vi "USB6343_Control_v1.4.vi"   [LabVIEW 2013]
uses:
  <vilib>/DAQmx/read.llb/DAQmx Read (Digital 1D Bool NChan 1Samp 1Line).vi
  <vilib>/DAQmx/read.llb/DAQmx Read (Analog 1D DBL NChan 1Samp).vi
  <vilib>/DAQmx/miscellaneous.llb/DAQmx Fill In Error Info.vi
  <vilib>/DAQmx/configure/timing.llb/DAQmx Timing (Implicit).vi
  offsets.vi
  <vilib>/DAQmx/write.llb/DAQmx Write (Digital 1D Bool NChan 1Samp 1Line).vi
  <vilib>/DAQmx/write.llb/DAQmx Write (Analog 1D DBL NChan 1Samp).vi
types:
  T1 = cluster{"source":string, "channel":i32, "old value":dbl, "new value":dbl, "on/off":bool}
  T2 = cluster{"cmd":string, "channel":i32, "value":dbl, "on/off":bool, "return value":refnum<vi>}
  T3 = cluster{"AI Task":refnum<k21>, "AO Task":refnum<k21>, "DO Task":refnum<k21>, "DI Task":refnum<k21>, "PWM x":refnum<k21>, "PWM y":refnum<k21>, "counter x":refnum<k21>, "counter y":refnum<k21>}
  T4 = cluster{"data":dbl, "data":dbl, "data":dbl, "data":dbl}
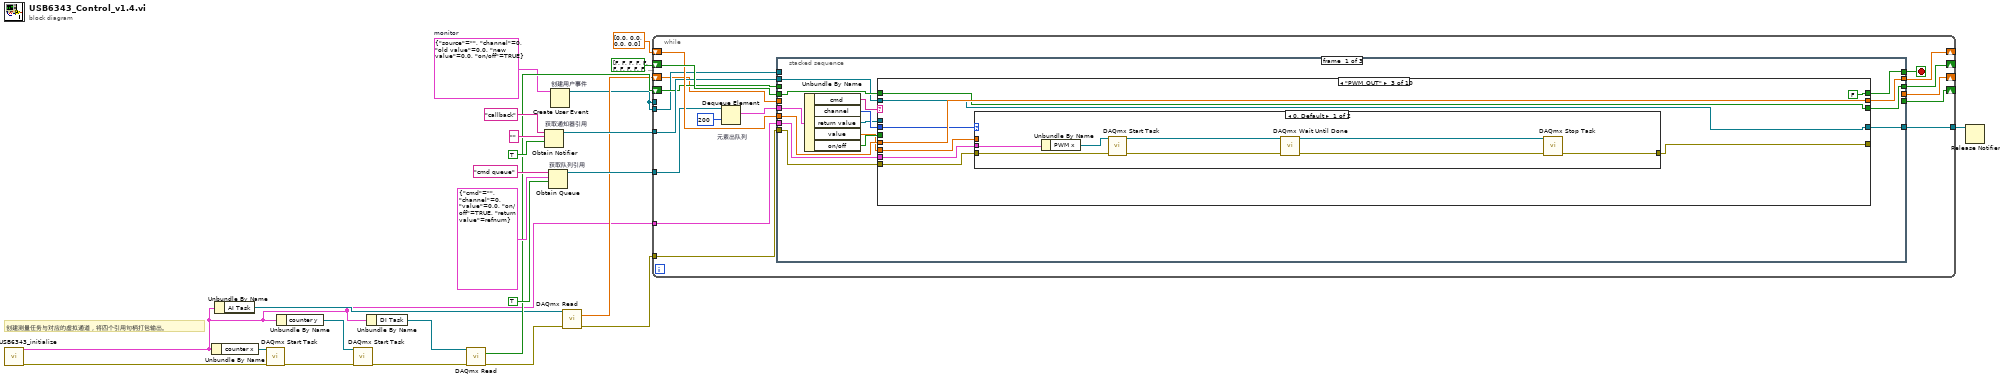
[diagram p0: block diagram]
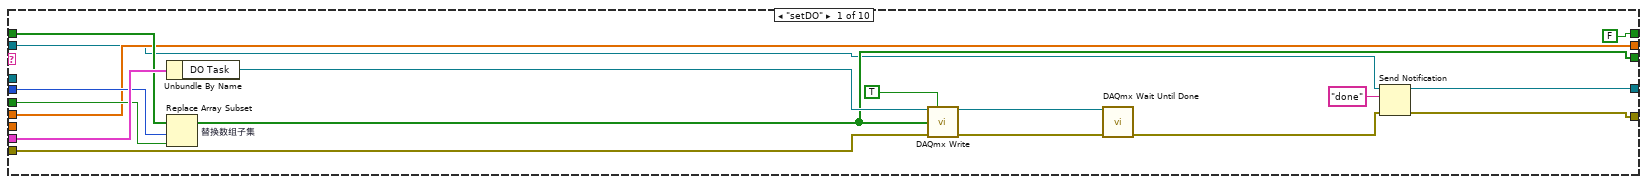
[diagram p2: hidden frame]
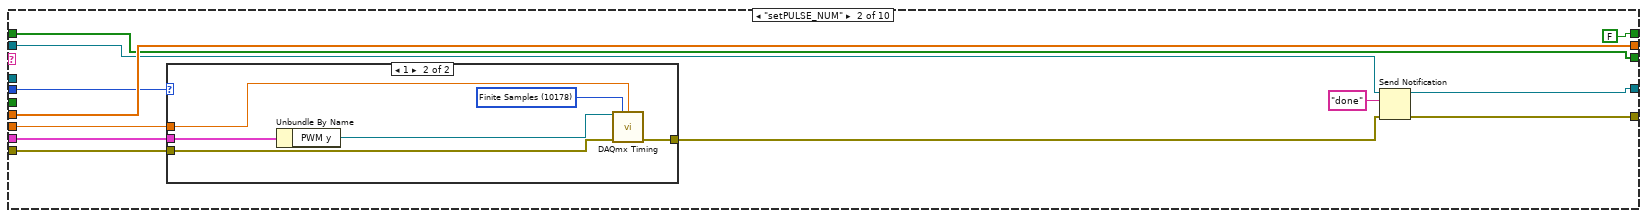
[diagram p3: hidden frame]
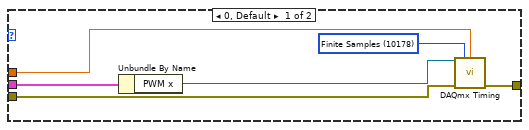
[diagram p4: hidden frame]
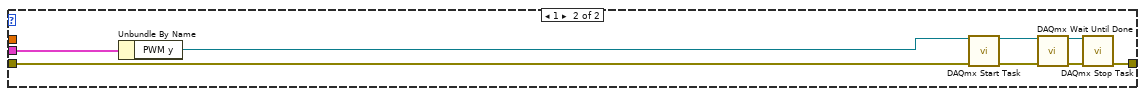
[diagram p5: hidden frame]
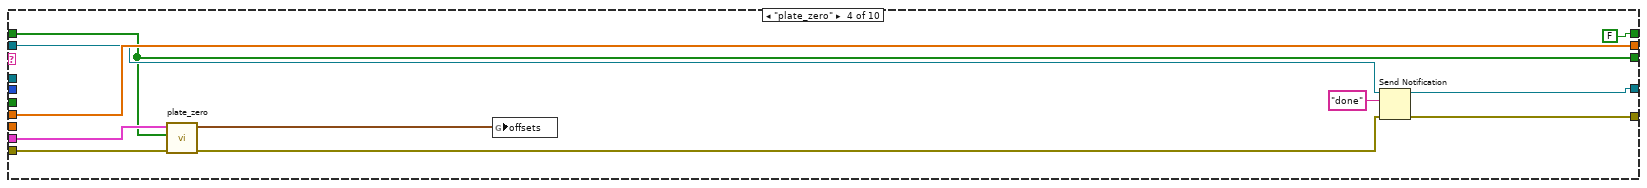
[diagram p6: hidden frame]
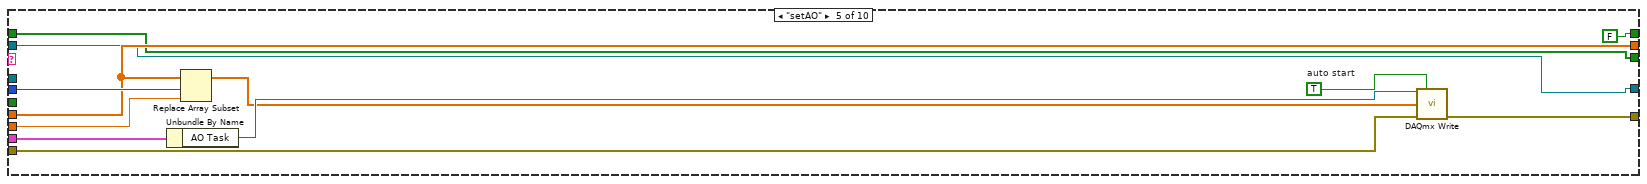
[diagram p7: hidden frame]
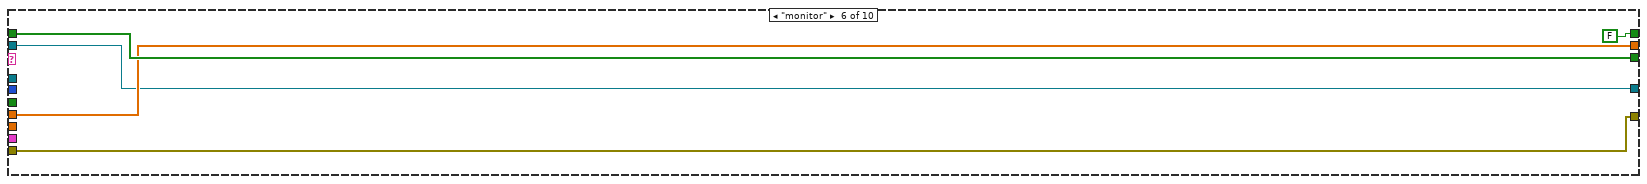
[diagram p8: hidden frame]
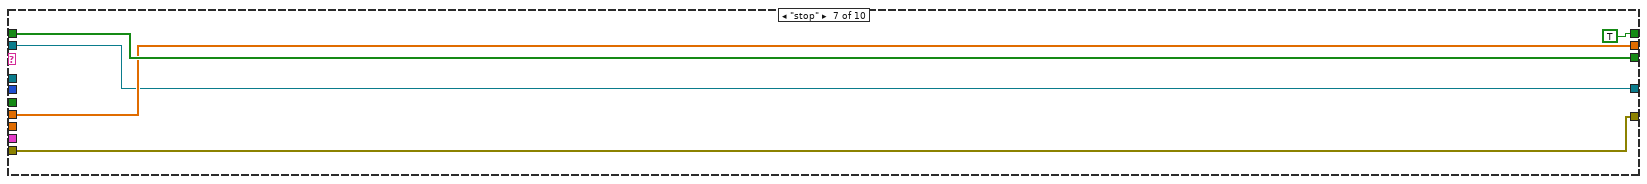
[diagram p9: hidden frame]
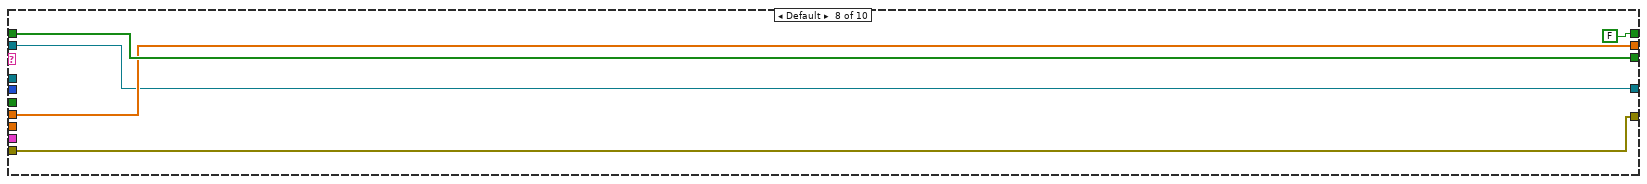
[diagram p10: hidden frame]
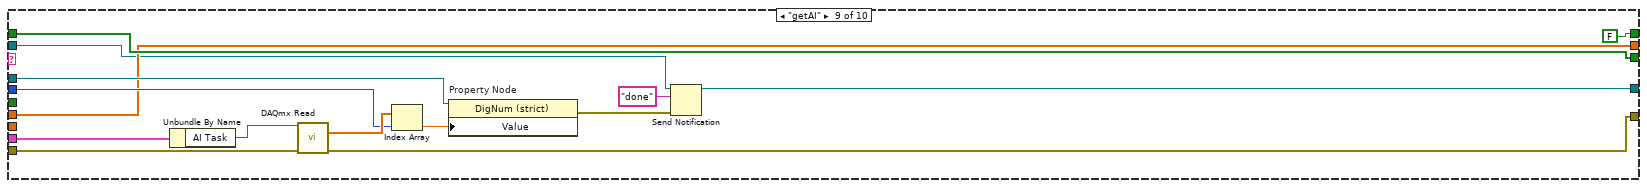
[diagram p11: hidden frame]
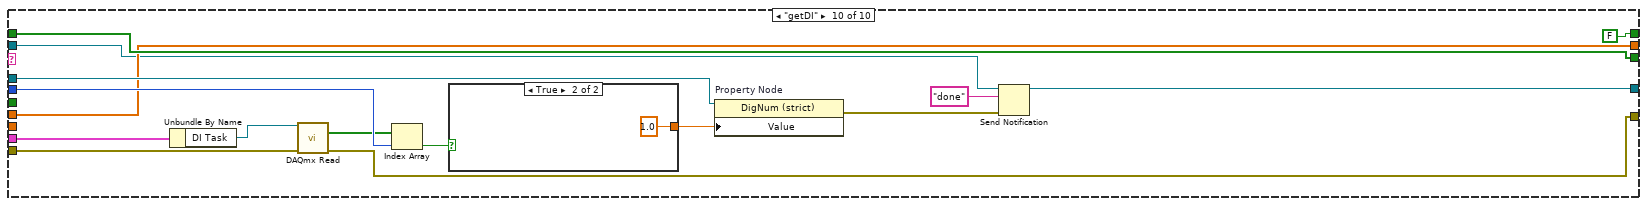
[diagram p12: hidden frame]
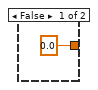
[diagram p13: hidden frame]
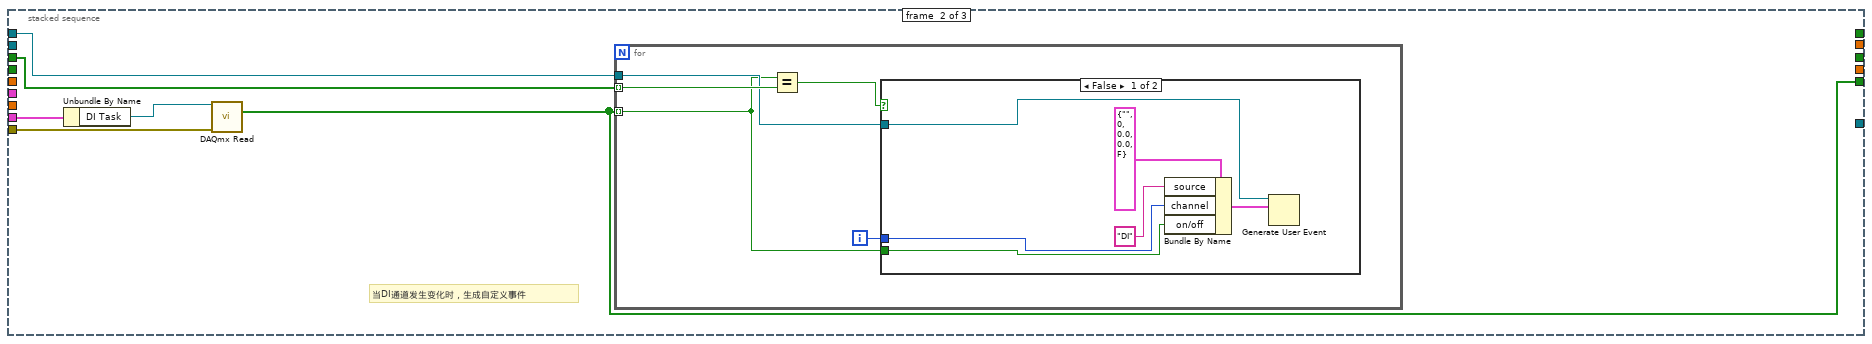
[diagram p14: hidden frame]
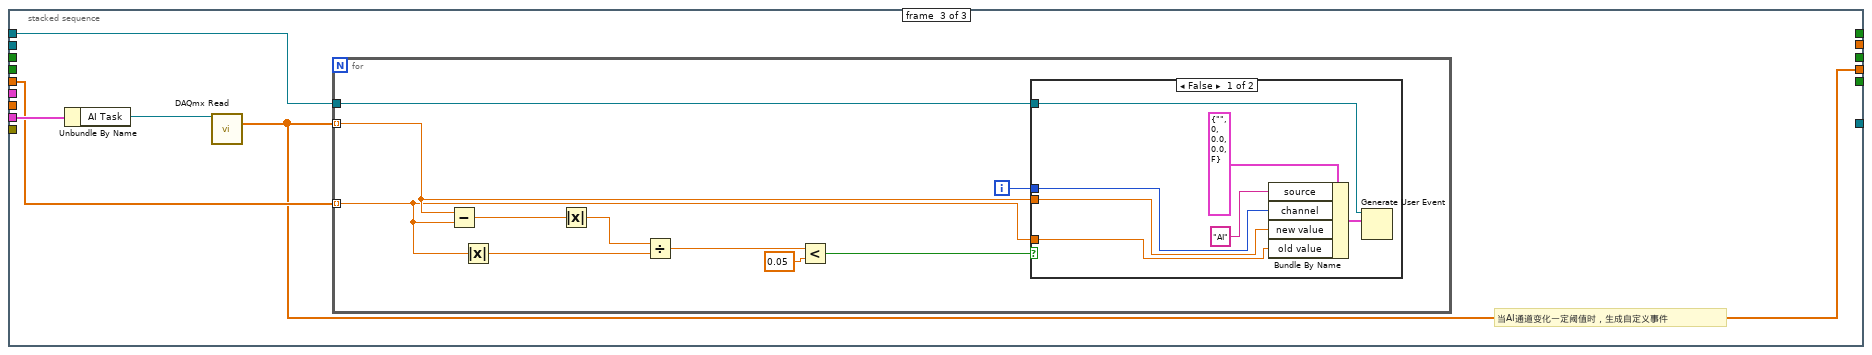
[diagram p16: hidden frame]
diagram:
  w8 = T1 {"source"="", "channel"=0, "old value"=0.0, "new value"=0.0, "on/off"=TRUE}  # monitor
  # "创建测量任务与对应的虚拟通道，将四个引用句柄打包输出。"
  n1 = call "USB6343_initialize.vi"() -> ("error out"=w5:errorcluster, "tasks"=w2:T3)  [unwired: 10 in]
  n2 = Unbundle By Name(w2) -> ("counter x"=w3:refnum<k21>)
  n3 = Unbundle By Name(w2) -> ("AI Task"=w10:refnum<k21>)
  n4 = call <vilib>:"DAQmx Start Task.vi"("task/channels in"=w3, "error in"=w5) -> ("error out"=w6:errorcluster)  [unwired: 12 in, 1 out]
  n5 = Unbundle By Name(w2) -> ("counter y"=w1:refnum<k21>)
  n6 = call <vilib>:"DAQmx Start Task.vi"("task/channels in"=w1, "error in"=w6) -> ("error out"=w4:errorcluster)  [unwired: 12 in, 1 out]
  n7 = Unbundle By Name(w2) -> ("DI Task"=w14:refnum<k21>)
  n8 = call-poly <vilib>:"DAQmx Read.vi"("task/channels in"=w14, "error in"=w4) -> ("data"=w13:bool[], "error out"=w12:errorcluster)  [unwired: 11 in, 1 out]
  n9 = Obtain Notifier "获取通知器引用"(name (unnamed)="callback" ("名称（未命名）"), notification data type="", create if not found? (T)=TRUE ("如未找到是否创建？(T)")) -> (notifier out=w17:refnum<notifier>)  [unwired: 1 in, 2 out]
  n10 = Obtain Queue "获取队列引用"(name (unnamed)="cmd queue" ("名称（未命名）"), element data type=T2 {"cmd"="", "channel"=0, "value"=0.0, "on/off"=TRUE, "return value"=refnum}, create if not found? (T)=TRUE ("如未找到是否创建？(T)")) -> (queue out=w21:refnum<queue>)  [unwired: 2 in, 2 out]
  n11 = Create User Event "创建用户事件"(user event datatype=w8) -> (user event=w7:refnum<user-event>)  [unwired: 1 in, 1 out]
  n12 = call-poly <vilib>:"DAQmx Read.vi"("task/channels in"=w10, "error in"=w12) -> ("data"=w9:dbl[], "error out"=w11:errorcluster)  [unwired: 11 in, 1 out]
  n13 = while {
    tunnel: w2 -> [w36]
    tunnel: w11 -> [w42]
    shift-right: [w40] -> _
    shift-left: bool[] [FALSE, FALSE, FALSE, FALSE, FALSE, FALSE, FALSE, FALSE, FALSE, FALSE, FALSE, FALSE, FALSE, FALSE, FALSE, FALSE] -> [w41]
    shift-right: [w37] -> _
    shift-left: dbl[] [0.0, 0.0, 0.0, 0.0] ("data") -> [w38]
    tunnel: w21 -> [w35]
    tunnel: w17 -> [w32]
    tunnel: [w31] -> w16
    shift-right: [w29] -> _
    shift-left: w13 -> [w30]
    shift-right: [w26] -> _
    shift-left: w9 -> [w27]
    tunnel: w7 -> [w28]
    tunnel: w7 -> [_]
    stop <- w39 stop-if-true
    n14 = Dequeue Element "元素出队列"(queue=w35, timeout in ms (-1)=200 ("超时毫秒(-1)")) -> (element=w34:T2)  [unwired: 1 in, 3 out]
    n15 = stacked-sequence {
      tunnel: w42 -> [w57 w198 _]
      tunnel: w41 -> [w56 _ _]
      tunnel: [w55 _ _] -> w40
      tunnel: [w54 _ _] -> w39
      tunnel: w38 -> [w53 _ _]
      tunnel: [w52 _ _] -> w37
      tunnel: w36 -> [w43 w200 w216]
      tunnel: w34 -> [w51 _ _]
      tunnel: w32 -> [w45 _ _]
      tunnel: [w44 _ _] -> w31
      tunnel: w30 -> [_ w197 _]
      tunnel: [_ w196 _] -> w29
      tunnel: w28 -> [_ w195 w212]
      tunnel: w27 -> [_ _ w214]
      tunnel: [_ _ w213] -> w26
      frame #0 {
        n16 = Unbundle By Name(w51) -> ("cmd"=w50:string, "channel"=w49:i32, "return value"=w48:refnum<vi>, "value"=w46:dbl, "on/off"=w47:bool)
        n17 = case shown="\"PWM_OUT\"" w50 {
          tunnel: w49 -> [w72 w75 w101 _ w144 _ _ _ w171 w190]
          tunnel: w43 -> [w74 w79 w104 w128 w146 _ _ _ w176 w192]
          tunnel: w57 -> [w66 w77 w102 w126 w138 w148 w153 w158 w173 w182]
          tunnel: w56 -> [w73 w80 w105 w127 w142 w151 w156 w161 w169 w189]
          tunnel: w47 -> [w71 _ _ _ _ _ _ _ _ _]
          tunnel: [w64 w80 w105 w127 w142 w151 w156 w161 w169 w189] -> w55
          tunnel: [FALSE FALSE FALSE FALSE FALSE FALSE TRUE FALSE FALSE FALSE] -> w54
          tunnel: w53 -> [w69 w85 w106 w133 w143 w150 w154 w159 w168 w188]
          tunnel: [w69 w85 w106 w133 w143 w150 w154 w159 w168 w188] -> w52
          tunnel: w48 -> [_ _ _ _ _ _ _ _ w174 w191]
          tunnel: [w68 w84 w100 w132 w135 w148 w153 w158 w166 w181] -> _
          tunnel: w46 -> [_ w78 w103 _ w137 _ _ _ _ _]
          tunnel: w45 -> [w59 w82 w99 w131 w136 w147 w152 w157 w163 w184]
          tunnel: [w58 w81 w99 w130 w136 w147 w152 w157 w162 w183] -> w44
          frame "setDO" {
            n18 = Unbundle By Name(w74) -> ("DO Task"=w65:refnum<k21>)
            n19 = Replace Array Subset "替换数组子集"(array=w73, new element=w71, index=w72) -> (w64:bool[])
            n20 = call-poly <vilib>:"DAQmx Write.vi"("task/channels in"=w65, "auto start"=TRUE, "data"=w64, "error in"=w66) -> ("task out"=w60:refnum<k21>, "error out"=w62:errorcluster)  [unwired: 9 in, 1 out]
            n21 = call <vilib>:"DAQmx Wait Until Done.vi"("task/channels in"=w60, "error in"=w62) -> ("error out"=w61:errorcluster)  [unwired: 12 in, 1 out]
            n22 = Send Notification(notification="done" ("通知"), notifier=w59, error in (no error)=w61) -> (notifier out=w58:refnum<notifier>, error out=w68:errorcluster)
          }
          frame "setPULSE_NUM" {
            n23 = case shown="1" w75 {
              tunnel: w79 -> [w92 w98]
              tunnel: w78 -> [w89 w95]
              tunnel: w77 -> [w88 w94]
              tunnel: [w87 w93] -> w76
              frame 0, Default {
                w90 = 10178 items=["Finite Samples"=10178, "Continuous Samples"=10123, "Hardware Timed Single Point"=12522] ("sample mode")
                n24 = Unbundle By Name(w92) -> ("PWM x"=w91:refnum<k21>)
                n25 = call-poly <vilib>:"DAQmx Timing.vi"("task/channels in"=w91, "sample mode"=w90, "samples per channel"=w89, "error in"=w88) -> ("error out"=w87:errorcluster)  [unwired: 10 in, 1 out]
              }
              frame 1 {
                w96 = 10178 items=["Finite Samples"=10178, "Continuous Samples"=10123, "Hardware Timed Single Point"=12522] ("sample mode")
                n26 = Unbundle By Name(w98) -> ("PWM y"=w97:refnum<k21>)
                n27 = call-poly <vilib>:"DAQmx Timing.vi"("task/channels in"=w97, "sample mode"=w96, "samples per channel"=w95, "error in"=w94) -> ("error out"=w93:errorcluster)  [unwired: 10 in, 1 out]
              }
            }
            n28 = Send Notification(notification="done" ("通知"), notifier=w82, error in (no error)=w76) -> (notifier out=w81:refnum<notifier>, error out=w84:errorcluster)
          }
          frame "PWM_OUT" {
            n29 = case shown="0, Default" w101 {
              tunnel: w104 -> [w115 w123]
              tunnel: w103 -> [_ _]
              tunnel: w102 -> [w113 w121]
              tunnel: [w108 w116] -> w100
              frame 0, Default {
                n30 = Unbundle By Name(w115) -> ("PWM x"=w114:refnum<k21>)
                n31 = call <vilib>:"DAQmx Start Task.vi"("task/channels in"=w114, "error in"=w113) -> ("task out"=w111:refnum<k21>, "error out"=w112:errorcluster)  [unwired: 12 in]
                n32 = call <vilib>:"DAQmx Wait Until Done.vi"("task/channels in"=w111, "error in"=w112) -> ("task out"=w109:refnum<k21>, "error out"=w110:errorcluster)  [unwired: 12 in]
                n33 = call <vilib>:"DAQmx Stop Task.vi"("task/channels in"=w109, "error in"=w110) -> ("error out"=w108:errorcluster)  [unwired: 12 in, 1 out]
              }
              frame 1 {
                n34 = Unbundle By Name(w123) -> ("PWM y"=w122:refnum<k21>)
                n35 = call <vilib>:"DAQmx Start Task.vi"("task/channels in"=w122, "error in"=w121) -> ("task out"=w119:refnum<k21>, "error out"=w120:errorcluster)  [unwired: 12 in]
                n36 = call <vilib>:"DAQmx Wait Until Done.vi"("task/channels in"=w119, "error in"=w120) -> ("task out"=w117:refnum<k21>, "error out"=w118:errorcluster)  [unwired: 12 in]
                n37 = call <vilib>:"DAQmx Stop Task.vi"("task/channels in"=w117, "error in"=w118) -> ("error out"=w116:errorcluster)  [unwired: 12 in, 1 out]
              }
            }
          }
          frame "plate_zero" {
            n38 = call "plate_zero.vi"("error in"=w126, "DO array"=w127, "tasks"=w128) -> ("error out"=w125:errorcluster, "offsets"=w124:T4)  [unwired: 7 in]
            n39 = global write "offsets.vi" "offsets"(w124) -> ()
            n40 = Send Notification(notification="done", notifier=w131, error in (no error)=w125) -> (notifier out=w130:refnum<notifier>, error out=w132:errorcluster)
          }
          frame "setAO" {
            w140 = TRUE  # auto start
            n41 = Unbundle By Name(w146) -> ("AO Task"=w145:refnum<k21>)
            n42 = Replace Array Subset(array=w143, new element=w137, index=w144) -> (w141:dbl[])
            n43 = call-poly <vilib>:"DAQmx Write.vi"("task/channels in"=w145, "auto start"=w140, "data"=w141, "error in"=w138) -> ("error out"=w135:errorcluster)  [unwired: 9 in, 2 out]
          }
          frame "monitor" {
          }
          frame "stop" {
          }
          frame Default {
          }
          frame "getAI" {
            n44 = Unbundle By Name(w176) -> ("AI Task"=w175:refnum<k21>)
            n45 = call-poly <vilib>:"DAQmx Read.vi"("task/channels in"=w175, "error in"=w173) -> ("data"=w172:dbl[], "error out"=w166:errorcluster)  [unwired: 11 in, 1 out]
            n46 = Index Array(array=w172, index=w171) -> (element=w170:dbl)
            n47 = property on="Property Node" class="DigNum (strict)"(reference=w174, "Value"=w170) -> (error out=w164:errorcluster)  [unwired: 1 in, 1 out]
            n48 = Send Notification(notification="done" ("通知"), notifier=w163, error in (no error)=w164) -> (notifier out=w162:refnum<notifier>)  [unwired: 1 out]
          }
          frame "getDI" {
            n49 = Unbundle By Name(w192) -> ("DI Task"=w180:refnum<k21>)
            n50 = call-poly <vilib>:"DAQmx Read.vi"("task/channels in"=w180, "error in"=w182) -> ("data"=w179:bool[], "error out"=w181:errorcluster)  [unwired: 11 in, 1 out]
            n51 = Index Array(array=w179, index=w190) -> (element=w178:bool)
            n52 = case shown="True" w178 {
              tunnel: [0.0 1.0] -> w177
              frame False {
              }
              frame True {
              }
            }
            n53 = property on="Property Node" class="DigNum (strict)"(reference=w191, "Value"=w177) -> (error out=w185:errorcluster)  [unwired: 1 in, 1 out]
            n54 = Send Notification(notification="done" ("通知"), notifier=w184, error in (no error)=w185) -> (notifier out=w183:refnum<notifier>)  [unwired: 1 out]
          }
        }
      }
      frame #1 {
        # "当DI通道发生变化时，生成自定义事件"
        n55 = Unbundle By Name(w200) -> ("DI Task"=w199:refnum<k21>)
        n56 = call-poly <vilib>:"DAQmx Read.vi"("task/channels in"=w199, "error in"=w198) -> ("data"=w196:bool[])  [unwired: 11 in, 2 out]
        n57 = for {
          tunnel: w196 -> [w201] mode=indexing
          tunnel: w197 -> [w205] mode=indexing
          tunnel: w195 -> [w202]
          i -> [w203]
          n58 = Equal?(x=w201, y=w205) -> (x = y?=w204:bool)
          n59 = case shown="False" w204 {
            tunnel: w203 -> [w208 _]
            tunnel: w202 -> [w211 _]
            tunnel: w201 -> [w207 _]
            frame False {
              n60 = Bundle By Name(cluster=T1 {"source"="", "channel"=0, "old value"=0.0, "new value"=0.0, "on/off"=FALSE} ("事件数据"), "source"="DI", "channel"=w208, "on/off"=w207) -> (w206:T1)
              n61 = Generate User Event(user event=w211, event data cluster=w206) -> ()  [unwired: 2 in, 2 out]
            }
            frame True {
            }
          }
        }
      }
      frame #2 {
        # "当AI通道变化一定阈值时，生成自定义事件"
        n62 = Unbundle By Name(w216) -> ("AI Task"=w215:refnum<k21>)
        n63 = call-poly <vilib>:"DAQmx Read.vi"("task/channels in"=w215) -> ("data"=w213:dbl[])  [unwired: 12 in, 2 out]
        n64 = for {
          tunnel: w213 -> [w218] mode=indexing
          tunnel: w214 -> [w217] mode=indexing
          tunnel: w212 -> [w220]
          i -> [w219]
          n65 = Subtract(x=w218, y=w217) -> (x-y=w226:dbl)
          n66 = Absolute Value(x=w217) -> (abs(x)=w224:dbl)
          n67 = Absolute Value(x=w226) -> (abs(x)=w225:dbl)
          n68 = Divide(x=w225, y=w224) -> (x/y=w223:dbl)
          n69 = Less?(x=w223, y=0.05) -> (x < y?=w221:bool)
          n70 = case shown="False" w221 {
            tunnel: w220 -> [w233 _]
            tunnel: w219 -> [w230 _]
            tunnel: w218 -> [w229 _]
            tunnel: w217 -> [w228 _]
            frame False {
              n71 = Bundle By Name(cluster=T1 {"source"="", "channel"=0, "old value"=0.0, "new value"=0.0, "on/off"=FALSE} ("事件数据"), "source"="AI", "channel"=w230, "new value"=w229, "old value"=w228) -> (w227:T1)
              n72 = Generate User Event(user event=w233, event data cluster=w227) -> ()  [unwired: 2 in, 2 out]
            }
            frame True {
            }
          }
        }
      }
    }
  }
  n73 = Release Notifier(notifier=w16) -> ()  [unwired: 2 in, 3 out]
